vi "TMP3x.vi"   [LabVIEW 2014, in "LMH-LINX.lvlib" / "TMP3x.lvlib"]
uses:
  <vilib>/MakerHub/LINX/Public/Sensors/Temperature/TMP3x/TMP3x.lvlib
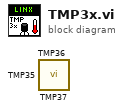
[diagram p0: block diagram]
diagram:
  n1 = call <vilib>:"TMP37.vi"() -> ()  [unwired: 9 in, 3 out]
  n2 = call <vilib>:"TMP36.vi"() -> ()  [unwired: 9 in, 3 out]
  n3 = call <vilib>:"TMP35.vi"() -> ()  [unwired: 9 in, 3 out]
